vi "dfd_Group Delay_Error.vi"(8 "error in (no error)":errorcluster, 10 "Coefficients":cluster{"r":dbl[], "theta":dbl[], "offset":dbl}, 11 "Design Info":T1={"p"=2, "freq grid"=[], "d"=[], "weight"=[], "Order"=0, "radius"=0.0}) -> (0 "error out":errorcluster, 1 "Error":dbl, 2 "Coefficients (dup)":cluster{"r":dbl[], "theta":dbl[], "offset":dbl}, 3 "Design Info (dup)":T1={"p"=2, "freq grid"=[], "d"=[], "weight"=[], "Order"=0, "radius"=0.0})   [LabVIEW 2017, in "NI_DigFilter_Design.lvlib"]
uses:
  <vilib>/addons/Digital Filter Design/NI_DigFilter_Design.lvlib
  <vilib>/addons/Digital Filter Design/_GroupDelay.llb/dfd_Group Delay_Design Info.ctl
  <vilib>/Analysis/NI_AALBase.lvlib
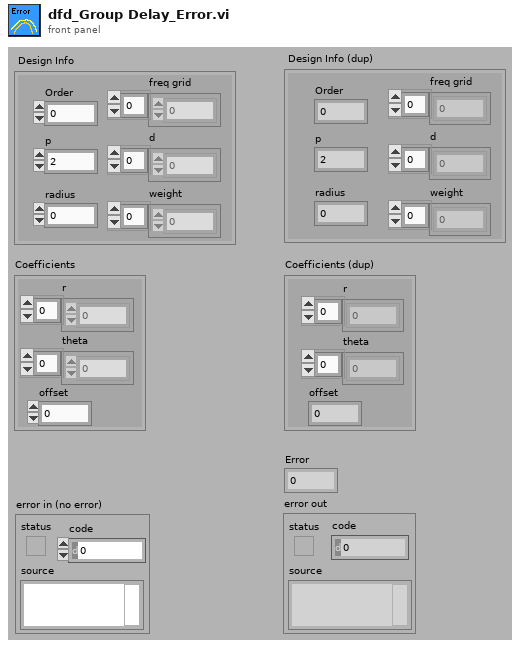
[diagram p1: front panel]
types:
  T1 = typedef "dfd_Group Delay_Design Info.ctl" = cluster{"p":i32, "freq grid":dbl[], "d":dbl[], "weight":dbl[], "Order":i32, "radius":dbl}
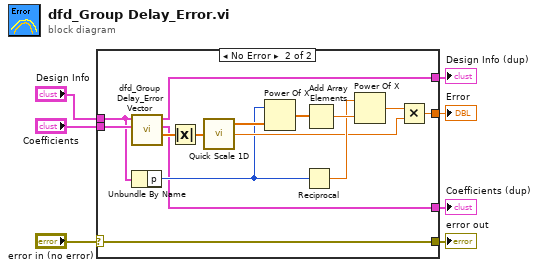
[diagram p0: block diagram]
diagram:
  n1 = case shown="No Error" "error in (no error)" {
    selector: "error in (no error)" -> [w8 w11]
    tunnel: [_ w20] -> w7
    tunnel: "Coefficients" -> [_ w16]
    tunnel: "Design Info" -> [_ w14]
    tunnel: [w8 w11] -> w5
    tunnel: [_ w10] -> w3
    tunnel: [_ w9] -> w1
    frame Error {
    }
    frame No Error {
      n2 = call <vilib>:"dfd_Group Delay_Error Vector.vi"("Coefficients"=w16, "Design Info"=w14) -> ("Error"=w15:dbl[], "Coefficients (dup)"=w9:cluster{"r":dbl[], "theta":dbl[], "offset":dbl}, "Design Info (dup)"=w10:T1)  [unwired: 7 out]
      n3 = Unbundle By Name(w14) -> ("p"=w13:i32)
      n4 = Absolute Value(x=w15) -> (abs(x)=w12:dbl[])
      n5 = call <vilib>:"Quick Scale 1D.vi"("X"=w12) -> ("Y[i]=X[i]/Max|X|"=w21:dbl[], "max|X|"=w18:dbl)  [unwired: 1 out]
      n6 = Power Of X(1:w21, 2:w13) -> (0:w17:dbl[])
      n7 = Reciprocal(x=w13) -> (1/x=w22:dbl)
      n8 = Add Array Elements(numeric array=w17) -> (sum=w23:dbl)
      n9 = Power Of X(1:w23, 2:w22) -> (0:w19:dbl)
      n10 = Multiply(x=w19, y=w18) -> (x*y=w20:dbl)
    }
  }
  "Error" <- w7
  "error out" <- w5
  "Design Info (dup)" <- w3
  "Coefficients (dup)" <- w1
